vi "OverlayResult.vi"(9 "DectectResult":variant, 10 "Algorithm":T3, 11 "Image":T2) -> (3 "Image Out":T2)   [LabVIEW 2019]
uses:
  Analysis/Controls/V_Analysis_Type.ctl
  <vilib>/vision/Image Controls.llb/IMAQ Image.ctl
  Analysis/Controls/ShapeDectect/V_ShapeDectectFinalResult.ctl
  Analysis/Controls/ShapeDectect/V_ShapeDectectResult.ctl
  Ctrl/ROIDataType.ctl
  Analysis/Controls/Color Pattern Match/Analysis Color Pattern Match Result.ctl
  Analysis/Controls/Geometric Match/Analysis_GeomatricPatternMatch_Result.ctl
  <vilib>/vision/Pattern Matching.llb/IMAQ GM Match Report.ctl
  Analysis/Controls/Area Check/Area Check_Result.ctl
panel:
  in  "Shapedectect Result Out":T1
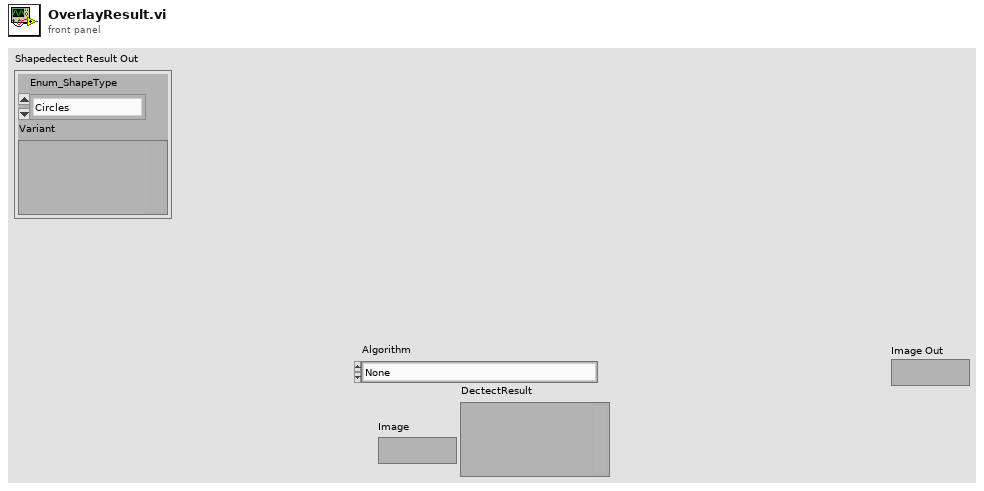
[diagram p1: front panel]
types:
  T1 = typedef "V_ShapeDectectFinalResult.ctl" = cluster{"Enum_ShapeType":enum16{"Circles", "Ellipses", "Lines", "Rectangles"}, "Variant":variant}
  T2 = typedef "IMAQ Image.ctl" = refnum<image>
  T3 = typedef "V_Analysis_Type.ctl" = enum16{"None", "C_Color Pattern Matching", "G_PatternMatching", "G_ShapeDectect", "G_GeometricMatch", "B_Area Check"}
  T4 = cluster{"Desired Font (Application)":enum16{"User-specified Font", "Application Font", "System Font", "Dialog Font"}, "[User-specified Font]":cluster{"Font Name":string, "Size":i16, "Strikeout?":bool, "Italic?":bool, "Underline?":bool, "Outline?":bool, "Shadow?":bool, "Bold?":bool, "Rotation Angle":dbl}, "Horizontal Alignment":i16, "Vertical Alignment":i16}
  T5 = typedef "V_ShapeDectectResult.ctl" = cluster{"ResultOut":variant, "DectectItem":i32, "Data out":T6, "ROIName":string}
  T6 = typedef "ROIDataType.ctl" = cluster{"Global Rectangle":i32[], "Contours":cluster{"Contour Type":u32, "ROI Type":u32, "Points":i32[]}[]}
  T7 = typedef "Analysis Color Pattern Match Result.ctl" = cluster{"Number of Matches":i32, "Matches out":cluster{"Position":cluster{"x":sgl, "y":sgl}, "Angle":sgl, "Scale":sgl, "Score":sgl, "Bounding Box":cluster{"x":sgl, "y":sgl}[]}[], "Calibrated Matches":cluster{"Position":cluster{"x":sgl, "y":sgl}, "Angle":sgl, "Scale":sgl, "Score":sgl, "Bounding Box":cluster{"x":sgl, "y":sgl}[]}[], "ROI Descriptor":T8, "ROIName":string}
  T8 = typedef "ROI Descriptor" = cluster{"Global Rectangle":i32[], "Contours":cluster{"ID":enum32{"External", "Internal"}, "Type":u32, "Coordinates":i32[]}[]}
  T9 = typedef "Analysis_GeomatricPatternMatch_Result.ctl" = cluster{"Number of Matches":i32, "Matches (pixel)":T10[], "Matches (real-world)":T10[], "Data out":T6, "ROIName":string}
  T10 = typedef "IMAQ GM Match Report.ctl" = cluster{"Position":cluster{"x":sgl, "y":sgl}, "Angle":sgl, "Scale":sgl, "Score":sgl, "Bounding Box":cluster{"x":sgl, "y":sgl}[], "Contrast Reversed":bool, "Occlusion %":sgl, "Template Target Curve Score":sgl, "Target Template Curve Score":sgl, "Correlation Score":sgl}
  T11 = typedef "Area Check_Result.ctl" = cluster{"AreaDataOut":cluster{"AreaDataOut":cluster{"Rectangle":T12, "Particle Measurements (Pixels)":dbl[][]}}[], "Percent":dbl[], "Item?":bool, "ROI":i32[]}
  T12 = typedef "IMAQ Rectangle" = cluster{"Left":i32, "Top":i32, "Right":i32, "Bottom":i32, "Rotation":dbl}
  T13 = cluster{"Position":cluster{"x":sgl, "y":sgl}, "Angle":sgl, "Scale":sgl, "Score":sgl, "Bounding Box":cluster{"x":sgl, "y":sgl}[]}[]
  T14 = enum16{"Circles", "Ellipses", "Lines", "Rectangles"}
  T15 = cluster{"Circles":cluster{"Position":cluster{"X":sgl, "Y":sgl}, "Radius":dbl, "Score":dbl}[], "Circles (Calibrated)":cluster{"Position":cluster{"X":sgl, "Y":sgl}, "Radius":dbl, "Score":dbl}[]}
  T16 = cluster{"Position":cluster{"X":sgl, "Y":sgl}, "Radius":dbl, "Score":dbl}[]
  T17 = cluster{"Pixel":cluster{"Position":cluster{"X":sgl, "Y":sgl}, "Angle":dbl, "Major Radius":dbl, "Minor Radius":dbl, "Score":dbl}[], "Ellipses (Calibrated)":cluster{"Position":cluster{"X":sgl, "Y":sgl}, "Orientation":dbl, "Major Radius":dbl, "Minor Radius":dbl, "Score":dbl}[]}
  T18 = cluster{"Position":cluster{"X":sgl, "Y":sgl}, "Angle":dbl, "Major Radius":dbl, "Minor Radius":dbl, "Score":dbl}[]
  T19 = cluster{"Lines":cluster{"Start Point":cluster{"X":sgl, "Y":sgl}, "End Point":cluster{"X":sgl, "Y":sgl}, "Length":dbl, "Angle":dbl, "Score":dbl}[], "Lines Calibrated":cluster{"Start Point":cluster{"X":sgl, "Y":sgl}, "End Point":cluster{"X":sgl, "Y":sgl}, "Length":dbl, "Orientation":dbl, "Score":dbl}[]}
  T20 = cluster{"Start Point":cluster{"X":sgl, "Y":sgl}, "End Point":cluster{"X":sgl, "Y":sgl}, "Length":dbl, "Angle":dbl, "Score":dbl}[]
  T21 = cluster{"Rectangles":cluster{"Corners":cluster{"X":sgl, "Y":sgl}[], "Angle":dbl, "Width":dbl, "Height":dbl, "Score":dbl}[], "Rectangles Calibrated":cluster{"Corners":cluster{"X":sgl, "Y":sgl}[], "Angle":dbl, "Width":dbl, "Height":dbl, "Score":dbl}[]}
  T22 = cluster{"Corners":cluster{"X":sgl, "Y":sgl}[], "Angle":dbl, "Width":dbl, "Height":dbl, "Score":dbl}[]
  T23 = cluster{"AreaDataOut":cluster{"Rectangle":T12, "Particle Measurements (Pixels)":dbl[][]}}[]
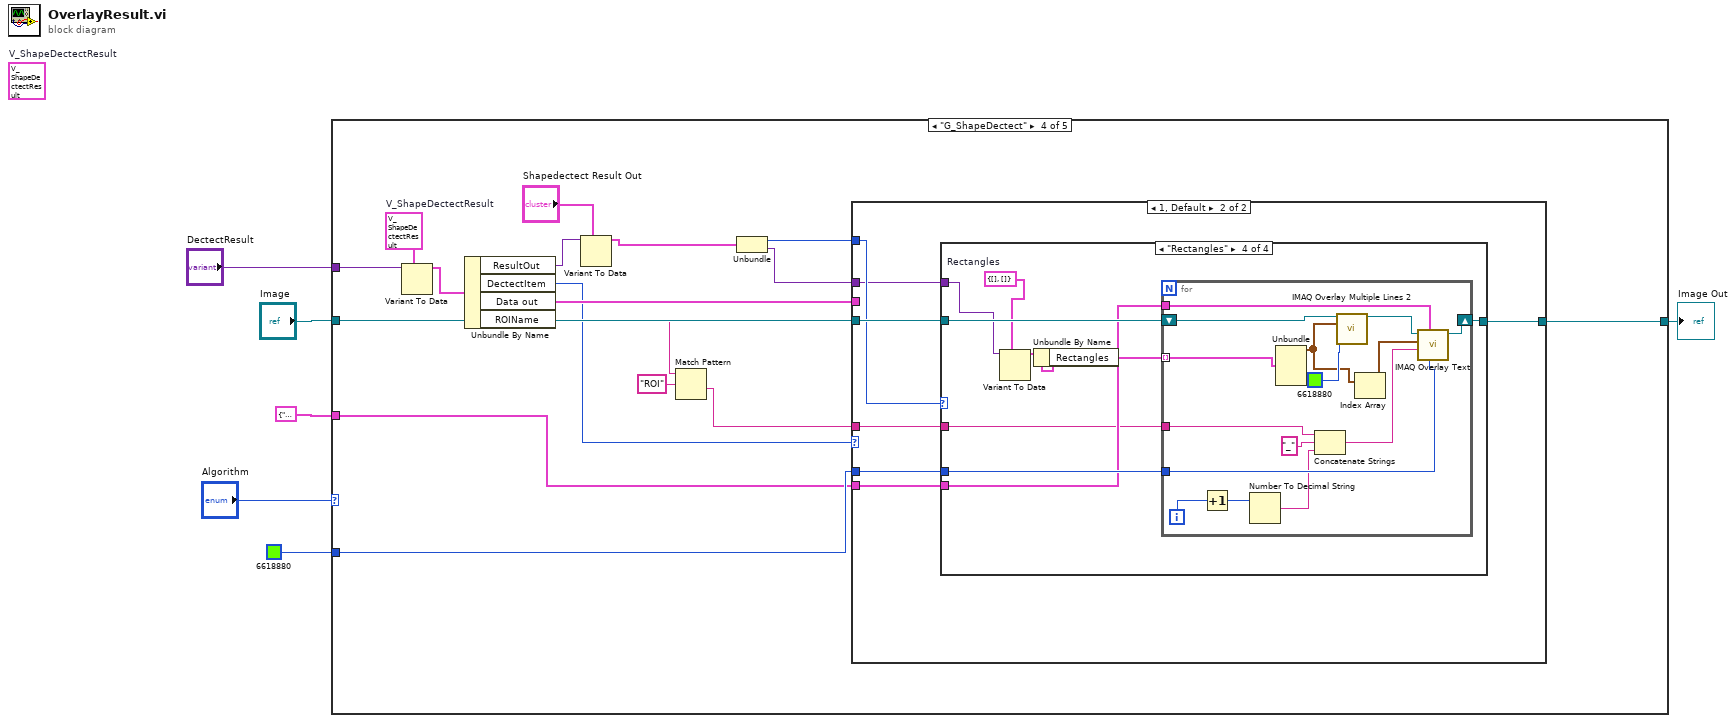
[diagram p0: block diagram]
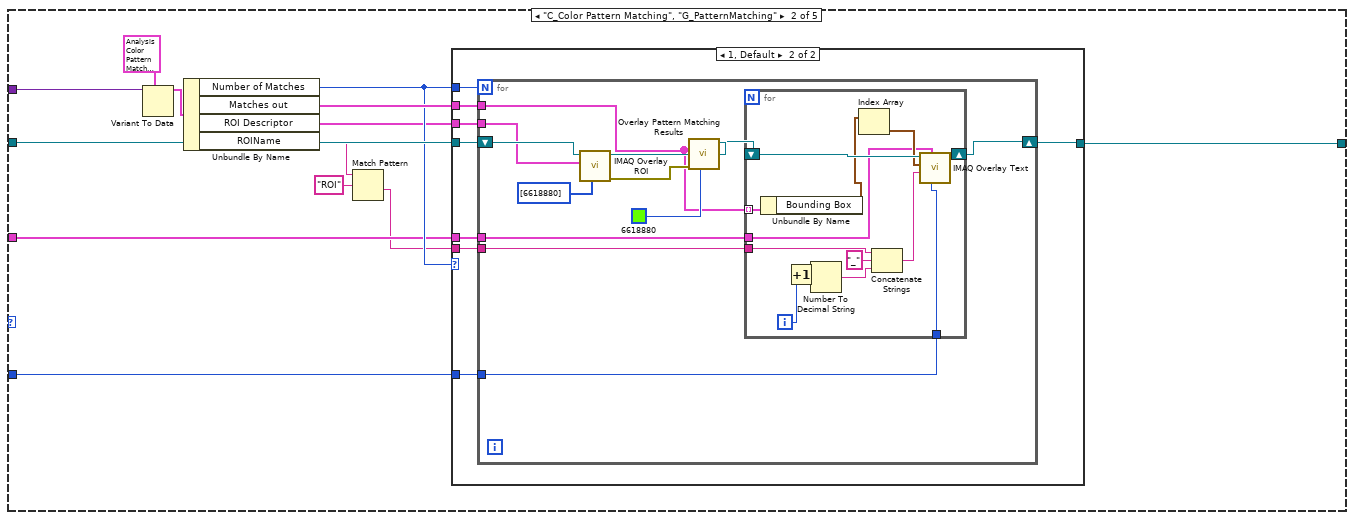
[diagram p3: hidden frame]
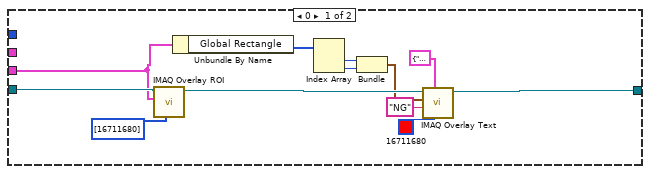
[diagram p4: hidden frame]
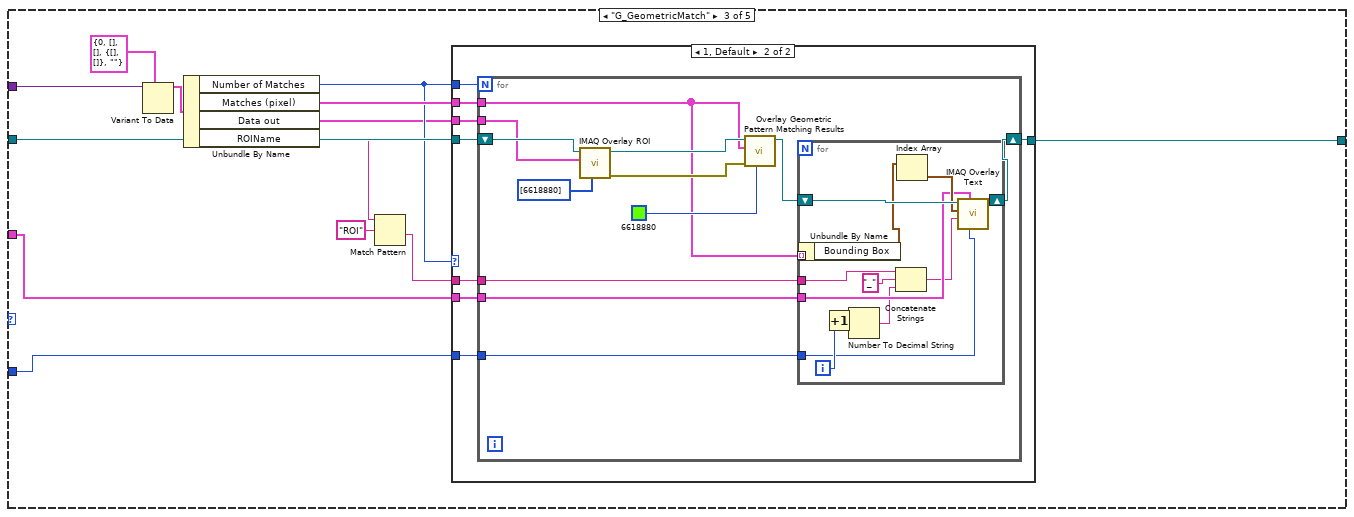
[diagram p5: hidden frame]
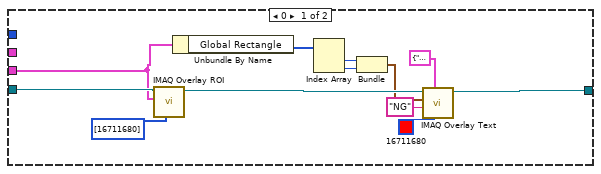
[diagram p6: hidden frame]
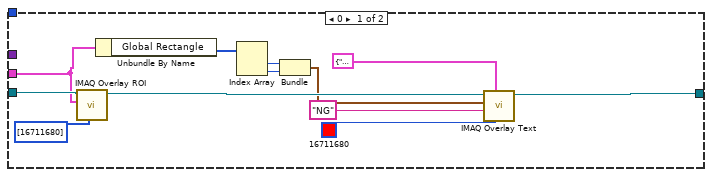
[diagram p7: hidden frame]
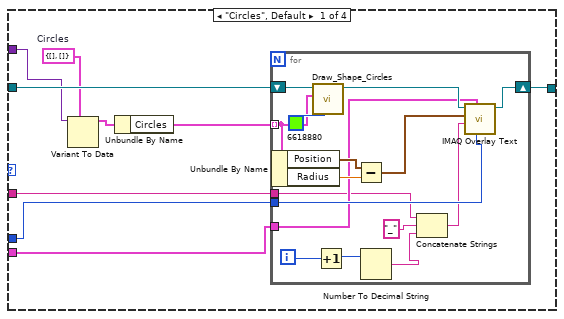
[diagram p8: hidden frame]
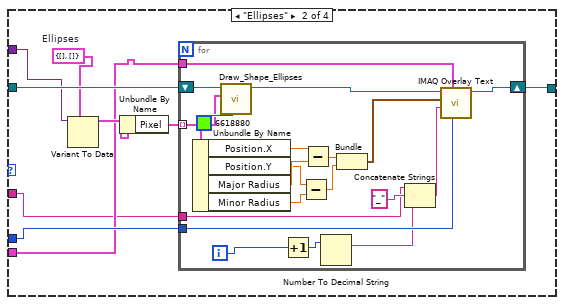
[diagram p9: hidden frame]
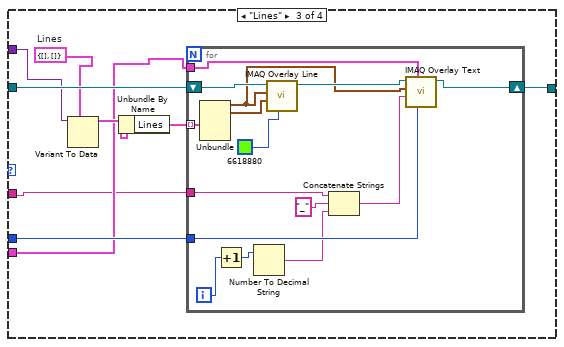
[diagram p10: hidden frame]
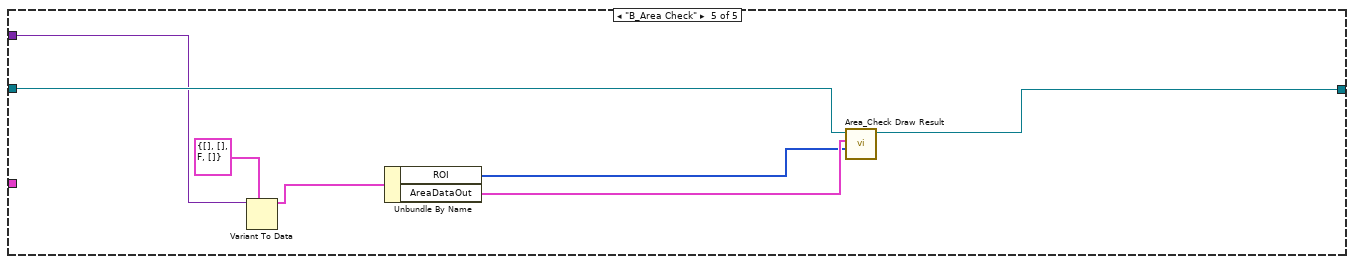
[diagram p11: hidden frame]
diagram:
  (unwired) T5 {"ResultOut"=variant, "DectectItem"=0, "Data out"={"Global Rectangle"=[], "Contours"=[]}, "ROIName"=""}  # V_ShapeDectectResult
  n1 = case shown="\"G_ShapeDectect\"" "Algorithm" {
    tunnel: "DectectResult" -> [_ w20 w78 w140 w265]
    tunnel: "Image" -> [w7 w17 w76 w138 w267]
    tunnel: [w7 w13 w72 w136 w268] -> w3
    tunnel: u32 6618880 ("Text Color (black)") -> [_ w12 w70 w128 _]
    tunnel: T4 {"Desired Font (Application)"=enum."User-specified Font", "[User-specified Font]"={"Font Name"="", "Size"=36, "Strikeout?"=FALSE, "Italic?"=FALSE, "Underline?"=FALSE, "Outline?"=FALSE, "Shadow?"=FALSE, "Bold?"=FALSE, "Rotation Angle"=0.0}, "Horizontal Alignment"=1, "Vertical Alignment"=0} ("Font, Size & Style") -> [_ w11 w69 w127 _]
    frame "None", Default {
    }
    frame "C_Color Pattern Matching", "G_PatternMatching" {
      n2 = Variant To Data(type=T7 {"Number of Matches"=0, "Matches out"=[{"Position"={"x"=123.0, "y"=0.0}, "Angle"=0.0, "Scale"=0.0, "Score"=0.0, "Bounding Box"=[]}, {"Position"={"x"=0.0, "y"=0.0}, "Angle"=0.0, "Scale"=0.0, "Score"=0.0, "Bounding Box"=[]}, {"Position"={"x"=0.0, "y"=0.0}, "Angle"=0.0, "Scale"=0.0, "Score"=0.0, "Bounding Box"=[]}, {"Position"={"x"=444.0, "y"=0.0}, "Angle"=0.0, "Scale"=0.0, "Score"=0.0, "Bounding Box"=[]}], "Calibrated Matches"=[], "ROI Descriptor"={"Global Rectangle"=[], "Contours"=[]}, "ROIName"=""} ("Color Pattern Matching"), Variant=w20) -> (data=w18:T7)  [unwired: 1 in, 1 out]
      n3 = Unbundle By Name(w18) -> ("Number of Matches"=w15:i32, "Matches out"=w16:T13, "ROI Descriptor"=w14:T8, "ROIName"=w10:string)
      n4 = Match Pattern(string=w10, regular expression="ROI") -> (after substring=w8:string)  [unwired: 1 in, 3 out]
      n5 = case shown="1, Default" w15 {
        tunnel: w15 -> [_ w40]
        tunnel: w17 -> [w32 w39]
        tunnel: w16 -> [_ w38]
        tunnel: w14 -> [w29 w37]
        tunnel: [w27 w36] -> w13
        tunnel: w12 -> [_ w35]
        tunnel: w11 -> [_ w34]
        tunnel: w8 -> [_ w33]
        frame 0 {
          n6 = call "IMAQ Overlay ROI"("Colors (Green)"=u32[] [16711680], "ROI Descriptor"=w29, "Image"=w32) -> ("Image Out"=w31:T2)  [unwired: 7 in, 1 out]
          n7 = Unbundle By Name(w29) -> ("Global Rectangle"=w28:i32[])
          n8 = Index Array(array=w28) -> (element #1=w25:i32, element #2=w26:i32)  [unwired: 2 in]
          n9 = Bundle(w25, w26) -> (w24:cluster{i32, i32})  [unwired: 1 in]
          n10 = call "IMAQ Overlay Text"("Text Color (black)"=u32 16711680, "Font, Size & Style"=T4 {"Desired Font (Application)"=enum."User-specified Font", "[User-specified Font]"={"Font Name"="", "Size"=24, "Strikeout?"=FALSE, "Italic?"=FALSE, "Underline?"=FALSE, "Outline?"=FALSE, "Shadow?"=FALSE, "Bold?"=FALSE, "Rotation Angle"=0.0}, "Horizontal Alignment"=0, "Vertical Alignment"=0}, "String"="NG", "Origin"=w24, "Image"=w31) -> ("Image Out"=w27:T2)  [unwired: 5 in, 1 out]
        }
        frame 1, Default {
          n11 = for {
            N: w40 -> [_]
            shift-right: [w44] -> w36
            shift-left: w39 -> [w51]
            tunnel: w38 -> [w45]
            tunnel: w37 -> [w50]
            tunnel: w35 -> [w43]
            tunnel: w34 -> [w42]
            tunnel: w33 -> [w41]
            n12 = call "IMAQ Overlay ROI"("Colors (Green)"=u32[] [6618880], "ROI Descriptor"=w50, "Image"=w51) -> ("error out"=w47:errorcluster, "Image Out"=w49:T2)  [unwired: 7 in]
            n13 = call "Overlay Pattern Matching Results.vi"("Color"=u32 6618880 ("Color (red)"), "error in"=w47, "Matches"=w45, "Image"=w49) -> ("Image Out"=w46:T2)  [unwired: 6 in, 1 out]
            n14 = for {
              shift-right: [w64] -> w44
              shift-left: w46 -> [w65]
              tunnel: w45 -> [w61] mode=indexing
              tunnel: w43 -> [w58]
              tunnel: w42 -> [w57]
              tunnel: w41 -> [w56]
              i -> [w63]
              n15 = Unbundle By Name(w61) -> ("Bounding Box"=w60:cluster{"x":sgl, "y":sgl}[])
              n16 = Increment(x=w63) -> (x+1=w62:i32)
              n17 = Number To Decimal String(number=w62) -> (decimal integer string=w54:string)  [unwired: 1 in]
              n18 = Index Array(array=w60) -> (element=w59:cluster{"x":sgl, "y":sgl})  [unwired: 1 in]
              n19 = Concatenate Strings(w56, "_" ("string"), w54) -> (w53:string)
              n20 = call "IMAQ Overlay Text"("Text Color (black)"=w58, "Font, Size & Style"=w57, "String"=w53, "Origin"=w59, "Image"=w65) -> ("Image Out"=w64:T2)  [unwired: 5 in, 1 out]
            }
          }
        }
      }
    }
    frame "G_GeometricMatch" {
      n21 = Variant To Data(type=T9 {"Number of Matches"=0, "Matches (pixel)"=[], "Matches (real-world)"=[], "Data out"={"Global Rectangle"=[], "Contours"=[]}, "ROIName"=""} ("GeomatricMatchResult"), Variant=w78) -> (data=w77:T9)  [unwired: 1 in, 1 out]
      n22 = Unbundle By Name(w77) -> ("Number of Matches"=w74:i32, "Matches (pixel)"=w75:T10[], "Data out"=w73:T6, "ROIName"=w67:string)
      n23 = Match Pattern(string=w67, regular expression="ROI") -> (after substring=w66:string)  [unwired: 1 in, 3 out]
      n24 = case shown="1, Default" w74 {
        tunnel: w74 -> [_ w98]
        tunnel: w76 -> [w90 w97]
        tunnel: w75 -> [_ w96]
        tunnel: w73 -> [w87 w95]
        tunnel: [w85 w94] -> w72
        tunnel: w70 -> [_ w93]
        tunnel: w69 -> [_ w92]
        tunnel: w66 -> [_ w91]
        frame 0 {
          n25 = call "IMAQ Overlay ROI"("Colors (Green)"=u32[] [16711680], "ROI Descriptor"=w87, "Image"=w90) -> ("Image Out"=w89:T2)  [unwired: 7 in, 1 out]
          n26 = Unbundle By Name(w87) -> ("Global Rectangle"=w86:i32[])
          n27 = Index Array(array=w86) -> (element #1=w83:i32, element #2=w84:i32)  [unwired: 2 in]
          n28 = Bundle(w83, w84) -> (w82:cluster{i32, i32})  [unwired: 1 in]
          n29 = call "IMAQ Overlay Text"("Text Color (black)"=u32 16711680, "Font, Size & Style"=T4 {"Desired Font (Application)"=enum."User-specified Font", "[User-specified Font]"={"Font Name"="", "Size"=24, "Strikeout?"=FALSE, "Italic?"=FALSE, "Underline?"=FALSE, "Outline?"=FALSE, "Shadow?"=FALSE, "Bold?"=FALSE, "Rotation Angle"=0.0}, "Horizontal Alignment"=0, "Vertical Alignment"=0}, "String"="NG", "Origin"=w82, "Image"=w89) -> ("Image Out"=w85:T2)  [unwired: 5 in, 1 out]
        }
        frame 1, Default {
          n30 = for {
            N: w98 -> [_]
            shift-right: [w103] -> w94
            shift-left: w97 -> [w109]
            tunnel: w96 -> [w102]
            tunnel: w95 -> [w108]
            tunnel: w93 -> [w101]
            tunnel: w92 -> [w100]
            tunnel: w91 -> [w99]
            n31 = call "IMAQ Overlay ROI"("Colors (Green)"=u32[] [6618880], "ROI Descriptor"=w108, "Image"=w109) -> ("error out"=w105:errorcluster, "Image Out"=w107:T2)  [unwired: 7 in]
            n32 = call "Overlay Geometric Pattern Matching Results.vi"("Color"=u32 6618880 ("Color (red)"), "error in"=w105, "Matches"=w102, "Image"=w107) -> ("Image Out"=w104:T2)  [unwired: 6 in, 1 out]
            n33 = for {
              shift-right: [w122] -> w103
              shift-left: w104 -> [w123]
              tunnel: w102 -> [w119] mode=indexing
              tunnel: w101 -> [w116]
              tunnel: w100 -> [w115]
              tunnel: w99 -> [w111]
              i -> [w121]
              n34 = Unbundle By Name(w119) -> ("Bounding Box"=w118:cluster{"x":sgl, "y":sgl}[])
              n35 = Increment(x=w121) -> (x+1=w120:i32)
              n36 = Number To Decimal String(number=w120) -> (decimal integer string=w113:string)  [unwired: 1 in]
              n37 = Concatenate Strings(w111, "_" ("string"), w113) -> (w112:string)
              n38 = Index Array(array=w118) -> (element=w117:cluster{"x":sgl, "y":sgl})  [unwired: 1 in]
              n39 = call "IMAQ Overlay Text"("Text Color (black)"=w116, "Font, Size & Style"=w115, "String"=w112, "Origin"=w117, "Image"=w123) -> ("Image Out"=w122:T2)  [unwired: 5 in, 1 out]
            }
          }
        }
      }
    }
    frame "G_ShapeDectect" {
      w135 = T5 {"ResultOut"=variant, "DectectItem"=0, "Data out"={"Global Rectangle"=[], "Contours"=[]}, "ROIName"=""}  # V_ShapeDectectResult
      n40 = Variant To Data(type=w135, Variant=w140) -> (data=w139:T5)  [unwired: 1 in, 1 out]
      n41 = Unbundle By Name(w139) -> ("ResultOut"=w133:variant, "DectectItem"=w134:i32, "Data out"=w137:T6, "ROIName"=w126:string)
      n42 = Variant To Data(type="Shapedectect Result Out", Variant=w133) -> (data=w131:T1)  [unwired: 1 in, 1 out]
      n43 = Match Pattern(string=w126, regular expression="ROI") -> (after substring=w125:string)  [unwired: 1 in, 3 out]
      n44 = Unbundle(w131) -> ("Enum_ShapeType"=w130:T14, "Variant"=w129:variant)
      n45 = case shown="1, Default" w134 {
        tunnel: w138 -> [w152 w159]
        tunnel: w137 -> [w149 _]
        tunnel: [w147 w157] -> w136
        tunnel: w130 -> [_ w158]
        tunnel: w129 -> [_ w156]
        tunnel: w128 -> [_ w155]
        tunnel: w127 -> [_ w154]
        tunnel: w125 -> [_ w153]
        frame 0 {
          n46 = call "IMAQ Overlay ROI"("Colors (Green)"=u32[] [16711680], "ROI Descriptor"=w149, "Image"=w152) -> ("Image Out"=w151:T2)  [unwired: 7 in, 1 out]
          n47 = Unbundle By Name(w149) -> ("Global Rectangle"=w148:i32[])
          n48 = Index Array(array=w148) -> (element #1=w145:i32, element #2=w146:i32)  [unwired: 2 in]
          n49 = Bundle(w145, w146) -> (w144:cluster{i32, i32})  [unwired: 1 in]
          n50 = call "IMAQ Overlay Text"("Text Color (black)"=u32 16711680, "Font, Size & Style"=T4 {"Desired Font (Application)"=enum."User-specified Font", "[User-specified Font]"={"Font Name"="", "Size"=24, "Strikeout?"=FALSE, "Italic?"=FALSE, "Underline?"=FALSE, "Outline?"=FALSE, "Shadow?"=FALSE, "Bold?"=FALSE, "Rotation Angle"=0.0}, "Horizontal Alignment"=0, "Vertical Alignment"=0}, "String"="NG", "Origin"=w144, "Image"=w151) -> ("Image Out"=w147:T2)  [unwired: 5 in, 1 out]
        }
        frame 1, Default {
          n51 = case shown="\"Rectangles\"" w158 {
            tunnel: w159 -> [w168 w193 w222 w246]
            tunnel: [w167 w192 w221 w245] -> w157
            tunnel: w156 -> [w165 w191 w220 w244]
            tunnel: w155 -> [w162 w187 w216 w240]
            tunnel: w154 -> [w161 w186 w215 w239]
            tunnel: w153 -> [w160 w185 w214 w238]
            frame "Circles", Default {
              w166 = T15 {"Circles"=[], "Circles (Calibrated)"=[]}  # Circles
              n52 = Variant To Data(type=w166, Variant=w165) -> (data=w164:T15)  [unwired: 1 in, 1 out]
              n53 = Unbundle By Name(w164) -> ("Circles"=w163:T16)
              n54 = for {
                shift-right: [w181] -> w167
                shift-left: w168 -> [w184]
                tunnel: w163 -> [w179] mode=indexing
                tunnel: w162 -> [w175]
                tunnel: w161 -> [w173]
                tunnel: w160 -> [w169]
                i -> [w180]
                n55 = Unbundle By Name(w179) -> ("Position"=w178:cluster{"X":sgl, "Y":sgl}, "Radius"=w177:dbl)
                n56 = call "Draw_Shape_Circles.vi"("Color"=u32 6618880, "Circle Descriptor"=w179, "Image"=w184) -> ("Image Out"=w182:T2)  [unwired: 7 in, 1 out]
                n57 = Increment(x=w180) -> (x+1=w174:i32)
                n58 = Subtract(x=w178, y=w177) -> (x-y=w176:cluster{"X":dbl, "Y":dbl})
                n59 = Number To Decimal String(number=w174) -> (decimal integer string=w171:string)  [unwired: 1 in]
                n60 = Concatenate Strings(w169, "_" ("string"), w171) -> (w170:string)
                n61 = call "IMAQ Overlay Text"("Text Color (black)"=w175, "Font, Size & Style"=w173, "String"=w170, "Origin"=w176, "Image"=w182) -> ("Image Out"=w181:T2)  [unwired: 5 in, 1 out]
              }
            }
            frame "Ellipses" {
              w188 = T17 {"Pixel"=[], "Ellipses (Calibrated)"=[]}  # Ellipses
              n62 = Variant To Data(type=w188, Variant=w191) -> (data=w190:T17)  [unwired: 1 in, 1 out]
              n63 = Unbundle By Name(w190) -> ("Pixel"=w189:T18)
              n64 = for {
                shift-right: [w208] -> w192
                shift-left: w193 -> [w213]
                tunnel: w189 -> [w207] mode=indexing
                tunnel: w187 -> [w199]
                tunnel: w186 -> [w198]
                tunnel: w185 -> [w194]
                i -> [w211]
                n65 = Unbundle By Name(w207) -> ("Position.X"=w206:sgl, "Position.Y"=w204:sgl, "Major Radius"=w205:dbl, "Minor Radius"=w203:dbl)
                n66 = call "Draw_Shape_Ellipses.vi"("Color"=u32 6618880, "Ellipse Descriptor"=w207, "Image"=w213) -> ("Image Out"=w209:T2)  [unwired: 7 in, 1 out]
                n67 = Increment(x=w211) -> (x+1=w210:i32)
                n68 = Subtract(x=w204, y=w203) -> (x-y=w201:dbl)
                n69 = Subtract(x=w206, y=w205) -> (x-y=w202:dbl)
                n70 = Number To Decimal String(number=w210) -> (decimal integer string=w196:string)  [unwired: 1 in]
                n71 = Bundle(w202, w201) -> (w200:cluster{dbl, dbl})  [unwired: 1 in]
                n72 = Concatenate Strings(w194, "_" ("string"), w196) -> (w195:string)
                n73 = call "IMAQ Overlay Text"("Text Color (black)"=w199, "Font, Size & Style"=w198, "String"=w195, "Origin"=w200, "Image"=w209) -> ("Image Out"=w208:T2)  [unwired: 5 in, 1 out]
              }
            }
            frame "Lines" {
              w217 = T19 {"Lines"=[], "Lines Calibrated"=[]}  # Lines
              n74 = Variant To Data(type=w217, Variant=w220) -> (data=w219:T19)  [unwired: 1 in, 1 out]
              n75 = Unbundle By Name(w219) -> ("Lines"=w218:T20)
              n76 = for {
                shift-right: [w231] -> w221
                shift-left: w222 -> [w237]
                tunnel: w218 -> [w235] mode=indexing
                tunnel: w216 -> [w228]
                tunnel: w215 -> [w227]
                tunnel: w214 -> [w223]
                i -> [w230]
                n77 = Unbundle(w235) -> ("Start Point"=w229:cluster{"X":sgl, "Y":sgl}, "End Point"=w234:cluster{"X":sgl, "Y":sgl})  [unwired: 3 out]
                n78 = Increment(x=w230) -> (x+1=w233:i32)
                n79 = Number To Decimal String(number=w233) -> (decimal integer string=w225:string)  [unwired: 1 in]
                n80 = call "IMAQ Overlay Line"("Color"=u32 6618880, "End Point"=w234, "Start Point"=w229, "Image"=w237) -> ("Image Out"=w232:T2)  [unwired: 6 in, 1 out]
                n81 = Concatenate Strings(w223, "_" ("string"), w225) -> (w224:string)
                n82 = call "IMAQ Overlay Text"("Text Color (black)"=w228, "Font, Size & Style"=w227, "String"=w224, "Origin"=w229, "Image"=w232) -> ("Image Out"=w231:T2)  [unwired: 5 in, 1 out]
              }
            }
            frame "Rectangles" {
              w241 = T21 {"Rectangles"=[], "Rectangles Calibrated"=[]}  # Rectangles
              n83 = Variant To Data(type=w241, Variant=w244) -> (data=w243:T21)  [unwired: 1 in, 1 out]
              n84 = Unbundle By Name(w243) -> ("Rectangles"=w242:T22)
              n85 = for {
                shift-right: [w255] -> w245
                shift-left: w246 -> [w261]
                tunnel: w242 -> [w259] mode=indexing
                tunnel: w240 -> [w252]
                tunnel: w239 -> [w251]
                tunnel: w238 -> [w247]
                i -> [w257]
                n86 = Increment(x=w257) -> (x+1=w258:i32)
                n87 = Number To Decimal String(number=w258) -> (decimal integer string=w248:string)  [unwired: 1 in]
                n88 = Unbundle(w259) -> ("Corners"=w254:cluster{"X":sgl, "Y":sgl}[])  [unwired: 4 out]
                n89 = Concatenate Strings(w247, "_" ("string"), w248) -> (w249:string)
                n90 = call "IMAQ Overlay Multiple Lines 2"("Image"=w261, "Line End Points"=w254, "Color"=u32 6618880) -> ("Image Out"=w256:T2)  [unwired: 11 in, 1 out]
                n91 = Index Array(array=w254) -> (element=w253:cluster{"X":sgl, "Y":sgl})  [unwired: 1 in]
                n92 = call "IMAQ Overlay Text"("Text Color (black)"=w252, "Font, Size & Style"=w251, "String"=w249, "Origin"=w253, "Image"=w256) -> ("Image Out"=w255:T2)  [unwired: 5 in, 1 out]
              }
            }
          }
        }
      }
    }
    frame "B_Area Check" {
      n93 = Variant To Data(type=T11 {"AreaDataOut"=[], "Percent"=[], "Item?"=FALSE, "ROI"=[]} ("cluster"), Variant=w265) -> (data=w264:T11)  [unwired: 1 in, 1 out]
      n94 = Unbundle By Name(w264) -> ("ROI"=w262:i32[], "AreaDataOut"=w263:T23)
      n95 = call "Area_Check Draw Result.vi"("ROI"=w262, "AreaDataOut"=w263, "Refnum in"=w267) -> ("Refnum out"=w268:T2)  [unwired: 7 in, 1 out]
    }
  }
  "Image Out" <- w3
